vi "PPMSDR - Sweep control._Anilvi.vi"(0 "Scan control":cluster{"Priority":u16, "Scan name":u16}[](array[cluster])=[{"Priority"=0, "Scan name"=4}, {"Priority"=3, "Scan name"=0}, {"Priority"=1, "Scan name"=0}, {"Priority"=3, "Scan name"=0}] {"Scan name" items=["OFF", "Vsg1", "Vsg2", "Vsgw", "Vbg", "Field", "Temp", "MW_freq", "MW_amplitude"]; "Priority" items=["Priority 0", "Priority 1", "Priority 2", "Priority 3", "Priority 4", "Priority 5"]}, 1 "Scan parameters":T2(array[cluster])=[{"DAQ Channel"=2, "Label"="\nappliedVsg=", "Scaled low"=-0.1, "Scaled high"=0.6, "Start"=-2.0, "End"=2.0, "Step"=0.02, "Scale?"=FALSE}, {"DAQ Channel"=3, "Label"="\nappliedTemp=", "Scaled low"=-0.175, "Scaled high"=0.775, "Start"=0.35, "End"=0.05, "Step"=0.05, "Scale?"=FALSE}, {"DAQ Channel"=3, "Label"="\nappliedVbg=", "Scaled low"=-0.11, "Scaled high"=0.31, "Start"=-60000.0, "End"=0.0, "Step"=5000.0, "Scale?"=FALSE}, {"DAQ Channel"=3, "Label"="\nappliedField=", "Scaled low"=-0.060000000000000005, "Scaled high"=0.14, "Start"=-55000.0, "End"=0.0, "Step"=5000.0, "Scale?"=FALSE}] {"Step" format="%#_6p"; "End" format="%#_6p"; "Start" format="%#_6p"; "Scaled high" format="%#_6p"; "Scaled low" format="%#_6p"}, 2 "Channels: AO 2":T1={"AO amp (V)"=[0.005, 0.0, 0.0, 0.0], "AO DC (V)"=[0.0, 0.0, 0.0, 0.0], "AO f (Hz)"=[0.25, 0.25, 0.25, 0.25], "AO phi (deg)"=[0.0, 0.0, 0.0, 0.0], "function"=[enum."Sawtooth Wave", enum."Sine Wave", enum."Sine Wave", enum."Sine Wave"]} {"AO DC (V)" format="%#_6p"; "AO amp (V)" format="%#_6p"}, 3 "Comments":string="Backgate sweep from -2 to 2V in 15mV step\n 60 mK\n\nI1=0\nI2: Left wire 3/5:  1m, 0.2, sawtooth wave\nV1: 4-terminal Right wire 1/28\nV2: Cross-Barrier 4/1", 4 "Experiment folder name":string="05-backgatesweep_I1V_test") -> ()   [LabVIEW 2013]
uses:
  <userlib>/Levylab/DAQ-Lockin-SubVI/Lockin-4461_MultiChannel - IV 3.0 globals.vi
  Labview_Local/Lockin-4461_Multiple Inputs and Outputs_KH Folder/P/users1/Joe/Lockin-4461_3.0 4461-4462 Multichannel Folder/DAQ-Lockin-SubVI/Lock-in Globles Multiple Inputs and Outputs.vi
panel:
  in  "Additional action (indexing priority)":u16[](array[ring])=[5, 5, 5, 5] items=["Clear DAQ Tasks", "Check Temperature", "Check Field Value", "Wait", "Temp Below X", "Do Nothing"]
  in  "Enum":enum16{"IV", "lockin", "IV/lockin continuous B"}(ring)
  in  "Number of IV curves":i32=1
  # "Instructions: \n1, you can put multiple scan names in one priority.\n2 OFF has to put in last priority"
  # "if you use the lockin\nprogram remember to\nset BG/SG parameters in\n'lockin_Vsg_multichannel.vi'"
  # "Make sure Lockin is in REMOTE mode"
  # "0"
  # "1"
  # "2"
  # "3"
  # "4"
  # "5"
  # "6"
  # "7"
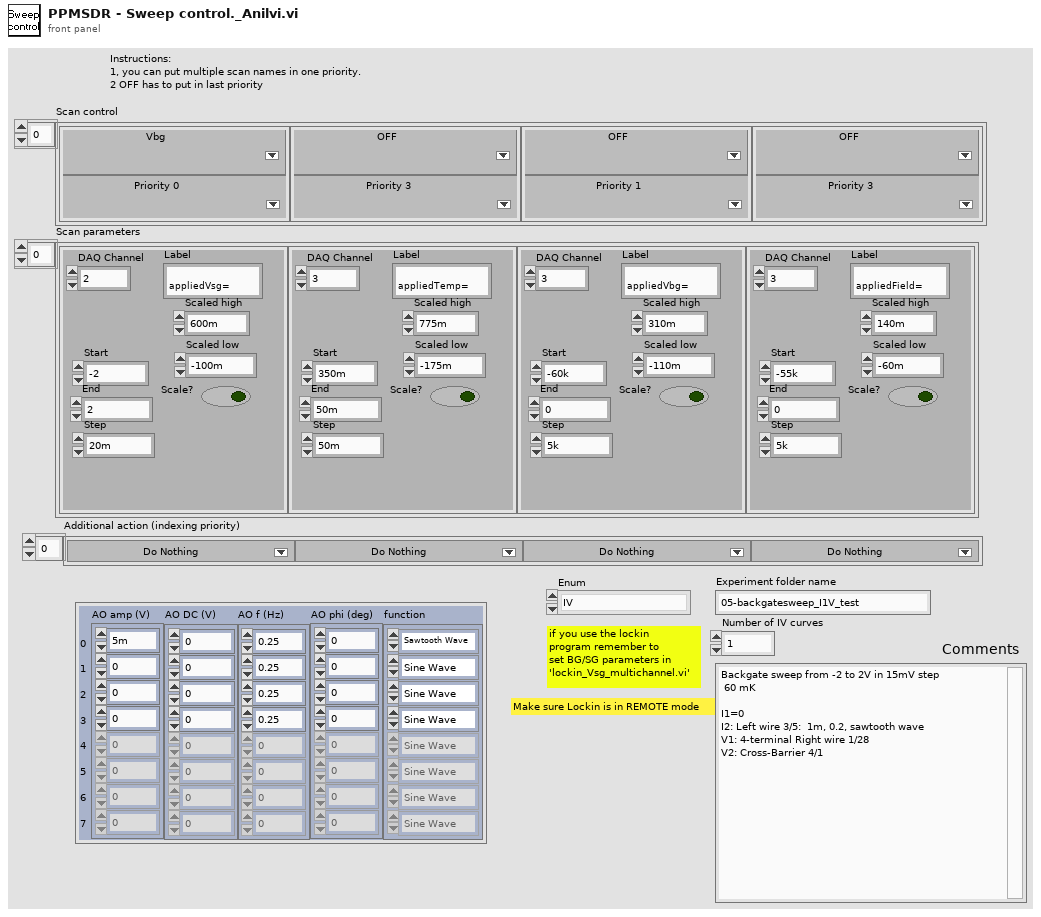
[diagram p1: front panel]
types:
  T1 = cluster{"AO amp (V)":dbl[], "AO DC (V)":dbl[], "AO f (Hz)":dbl[], "AO phi (deg)":dbl[], "function":enum16{"Sine Wave", "Triangle Wave", "Square Wave", "Sawtooth Wave"}[]}
  T2 = cluster{"DAQ Channel":i32, "Label":string, "Scaled low":dbl, "Scaled high":dbl, "Start":dbl, "End":dbl, "Step":dbl, "Scale?":bool}[]
  T3 = cluster{cluster{"DAQ Channel":i32, "Label":string, "Scaled low":dbl, "Scaled high":dbl, "Start":dbl, "End":dbl, "Step":dbl, "Scale?":bool}[]}[]
  T4 = cluster{cluster{"Priority":u16, "Scan name":u16}[]}[]
  T5 = cluster{cluster{"DAQ Channel":i32, "Label":string, "Scaled low":dbl, "Scaled high":dbl, "Start":dbl, "End":dbl, "Step":dbl, "Scale?":bool}[]}
  T6 = cluster{cluster{"Priority":u16, "Scan name":u16}[]}
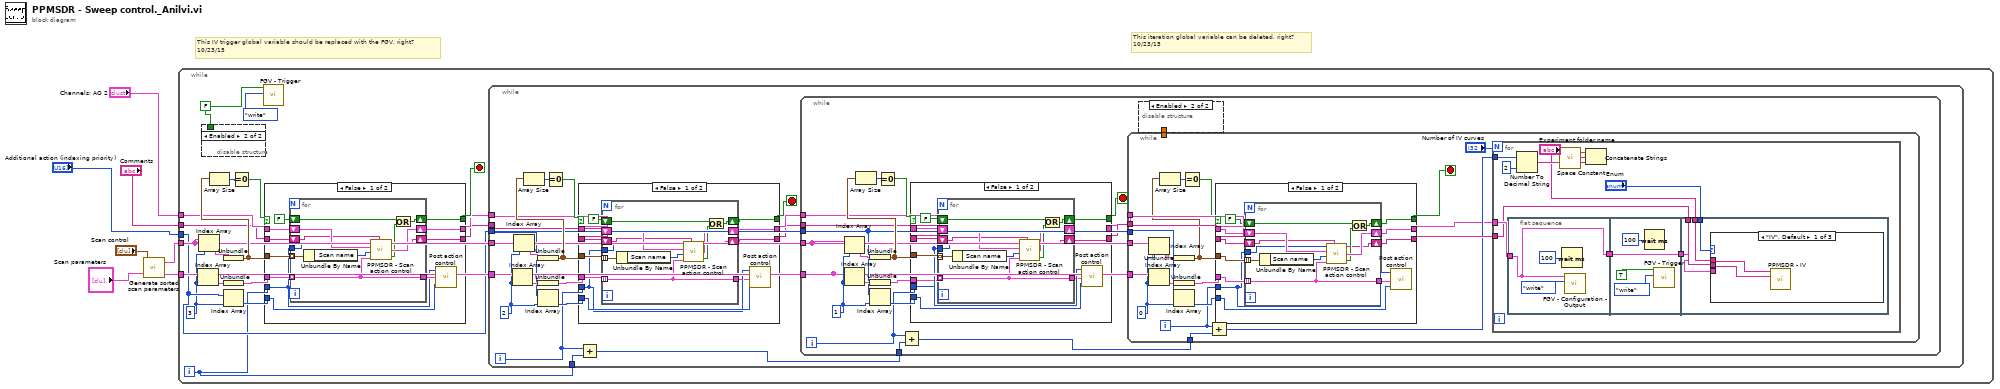
[diagram p0: block diagram]
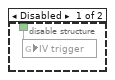
[diagram p2: hidden frame]
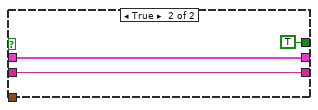
[diagram p3: hidden frame]
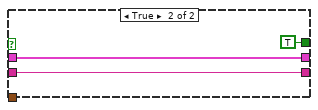
[diagram p4: hidden frame]
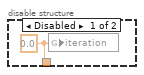
[diagram p5: hidden frame]
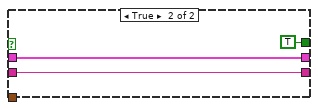
[diagram p6: hidden frame]
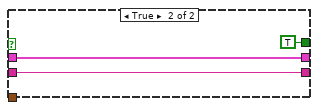
[diagram p7: hidden frame]
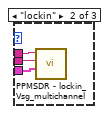
[diagram p8: hidden frame]
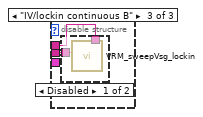
[diagram p9: hidden frame]
diagram:
  # "This IV trigger global variable should be replaced with the FGV, right?\n10/23/15"
  # "This iteration global variable can be deleted, right?\n10/23/15"
  n1 = call <userlib>:"Generate sorted scan parameters.vi"("Scan parameters"="Scan parameters", "Scan control"="Scan control") -> ("Sorted scan parameters"=w3:T3, "Sorted scan control"=w4:T4)
  n2 = while {
    tunnel: "Comments" -> [w14]
    tunnel: "Channels: AO 2" -> [w15]
    tunnel: w3 -> [w21]
    tunnel: w4 -> [w20]
    tunnel: "Additional action (indexing priority)" -> [w16]
    i -> [w10]
    stop <- w18 stop-if-true
    w8 = FALSE
    w11 = 3
    n3 = Index Array(array=w21, index=w11) -> (element=w22:T5)
    n4 = Index Array(array=w20, index=w11) -> (element=w19:T6)
    n5 = disable-structure shown="Enabled" {
      disable-tunnel: w8 -> [w27 _]
      frame Disabled {
        n6 = global write "Lock-in Globles Multiple Inputs and Outputs.vi" "IV trigger"(w27) -> ()
      }
      frame Enabled {
      }
    }
    n7 = Unbundle(w19) -> (w24:cluster{"Priority":u16, "Scan name":u16}[])
    n8 = Array Size(array=w24) -> (size(s)=w25:i32)
    n9 = Unbundle(w22) -> (w23:T2)
    n10 = Index Array(array=w16, index=w11) -> (element=w17:u16)
    n11 = Equal To 0?(x=w25) -> (x = 0?=w26:bool)
    n12 = call "FGV - Trigger.vi"("Function"=enum16{"write", "read"}."write", "Trigger"=w8) -> ()  [unwired: 4 in, 2 out]
    n13 = case shown="False" w26 {
      tunnel: w23 -> [w38 _]
      tunnel: [w37 w51] -> w13
      tunnel: [w36 w50] -> w12
      tunnel: [w30 TRUE ("Stop?")] -> w18
      tunnel: w24 -> [w35 _]
      tunnel: w10 -> [w32 _]
      tunnel: w17 -> [w33 _]
      tunnel: w15 -> [w29 w51]
      tunnel: w14 -> [w28 w50]
      frame False {
        n14 = for {
          tunnel: w35 -> [w49] mode=indexing
          tunnel: w38 -> [w46] mode=indexing
          tunnel: w32 -> [w43]
          shift-right: [w41] -> w37
          shift-left: w29 -> [w44]
          shift-right: [w39] -> w36
          shift-left: w28 -> [w42]
          tunnel: [w46] -> w34
          shift-right: [w47] -> w30
          shift-left: FALSE -> [w48]
          n15 = Unbundle By Name(w49) -> ("Scan name"=w45:u16)
          n16 = call <userlib>:"PPMSDR - Scan action control.vi"("Index"=w43, "Channels: AO"=w44, "Scan control"=w45, "Scan Parameters"=w46, "Comments"=w42) -> ("Comments out"=w39:string, "Channels: AO 2"=w41:T1, "Stop?"=w40:bool)
          n17 = Or(x=w48, y=w40) -> (x .or. y?=w47:bool)
        }
        n18 = call <userlib>:"Post action control.vi"("Action"=w33, "Scan Parameters"=w34, "Index"=w32) -> ()  [unwired: 1 out]
      }
      frame True {
      }
    }
    n19 = while {
      tunnel: w21 -> [w64]
      tunnel: w20 -> [w63]
      tunnel: w16 -> [w62]
      tunnel: w12 -> [w61]
      tunnel: w13 -> [w60]
      tunnel: w10 -> [w54]
      i -> [w55]
      stop <- w59 stop-if-true
      w56 = 2
      n20 = Index Array(array=w64, index=w56) -> (element=w70:T5)
      n21 = Index Array(array=w63, index=w56) -> (element=w71:T6)
      n22 = Unbundle(w71) -> (w68:cluster{"Priority":u16, "Scan name":u16}[])
      n23 = Array Size(array=w68) -> (size(s)=w66:i32)
      n24 = Unbundle(w70) -> (w69:T2)
      n25 = Index Array(array=w62, index=w56) -> (element=w67:u16)
      n26 = Equal To 0?(x=w66) -> (x = 0?=w65:bool)
      n27 = case shown="False" w65 {
        tunnel: w69 -> [w77 _]
        tunnel: w60 -> [w80 w96]
        tunnel: w61 -> [w79 w95]
        tunnel: [w74 w96] -> w58
        tunnel: [w73 w95] -> w57
        tunnel: [w75 TRUE ("Stop?")] -> w59
        tunnel: w68 -> [w78 _]
        tunnel: w55 -> [w76 _]
        tunnel: w67 -> [w82 _]
        frame False {
          n28 = for {
            tunnel: w78 -> [w93] mode=indexing
            tunnel: w77 -> [w90] mode=indexing
            tunnel: w76 -> [w87]
            shift-right: [w85] -> w74
            shift-left: w80 -> [w88]
            shift-right: [w83] -> w73
            shift-left: w79 -> [w86]
            tunnel: [w90] -> w72
            shift-right: [w91] -> w75
            shift-left: FALSE -> [w92]
            n29 = Unbundle By Name(w93) -> ("Scan name"=w89:u16)
            n30 = call <userlib>:"PPMSDR - Scan action control.vi"("Index"=w87, "Channels: AO"=w88, "Scan control"=w89, "Scan Parameters"=w90, "Comments"=w86) -> ("Comments out"=w83:string, "Channels: AO 2"=w85:T1, "Stop?"=w84:bool)
            n31 = Or(x=w92, y=w84) -> (x .or. y?=w91:bool)
          }
          n32 = call <userlib>:"Post action control.vi"("Action"=w82, "Scan Parameters"=w72, "Index"=w76) -> ()  [unwired: 1 out]
        }
        frame True {
        }
      }
      n33 = Add(x=w55, y=w54) -> (x+y=w53:i32)
      n34 = while {
        tunnel: w58 -> [w98]
        tunnel: w57 -> [w108]
        tunnel: w63 -> [w107]
        tunnel: w64 -> [w97]
        tunnel: w62 -> [w106]
        tunnel: w53 -> [w100]
        i -> [w101]
        stop <- w103 stop-if-true
        w102 = 1
        n35 = Index Array(array=w107, index=w102) -> (element=w109:T6)
        n36 = Index Array(array=w97, index=w102) -> (element=w110:T5)
        n37 = Unbundle(w109) -> (w112:cluster{"Priority":u16, "Scan name":u16}[])
        n38 = Array Size(array=w112) -> (size(s)=w114:i32)
        n39 = Unbundle(w110) -> (w111:T2)
        n40 = Index Array(array=w106, index=w102) -> (element=w113:u16)
        n41 = Equal To 0?(x=w114) -> (x = 0?=w115:bool)
        n42 = Add(x=w101, y=w100) -> (x+y=w99:i32)
        n43 = case shown="False" w115 {
          tunnel: w111 -> [w122 _]
          tunnel: w98 -> [w126 w142]
          tunnel: w108 -> [w125 w141]
          tunnel: [w120 w142] -> w104
          tunnel: [w119 w141] -> w105
          tunnel: [w121 TRUE ("Stop?")] -> w103
          tunnel: w112 -> [w124 _]
          tunnel: w101 -> [w123 _]
          tunnel: w113 -> [w128 _]
          frame False {
            n44 = for {
              tunnel: w124 -> [w139] mode=indexing
              tunnel: w122 -> [w136] mode=indexing
              tunnel: w123 -> [w133]
              shift-right: [w131] -> w120
              shift-left: w126 -> [w134]
              shift-right: [w129] -> w119
              shift-left: w125 -> [w132]
              tunnel: [w136] -> w118
              shift-right: [w137] -> w121
              shift-left: FALSE -> [w138]
              n45 = Unbundle By Name(w139) -> ("Scan name"=w135:u16)
              n46 = call <userlib>:"PPMSDR - Scan action control.vi"("Index"=w133, "Channels: AO"=w134, "Scan control"=w135, "Scan Parameters"=w136, "Comments"=w132) -> ("Comments out"=w129:string, "Channels: AO 2"=w131:T1, "Stop?"=w130:bool)
              n47 = Or(x=w138, y=w130) -> (x .or. y?=w137:bool)
            }
            n48 = call <userlib>:"Post action control.vi"("Action"=w128, "Scan Parameters"=w118, "Index"=w123) -> ()  [unwired: 1 out]
          }
          frame True {
          }
        }
        n49 = disable-structure shown="Enabled" {
          disable-tunnel: [w117 _] -> w116
          frame Disabled {
            w117 = 0.0 ("iteration")
            n50 = global write "Lockin-4461_MultiChannel - IV 3.0 globals.vi" "iteration"(w117) -> ()
          }
          frame Enabled {
          }
        }
        n51 = while {
          tunnel: w107 -> [w161]
          tunnel: w97 -> [w160]
          tunnel: w104 -> [w156]
          tunnel: w105 -> [w155]
          tunnel: w106 -> [w151]
          tunnel: w116 -> [_]
          tunnel: w99 -> [w145]
          i -> [w146]
          stop <- w153 stop-if-true
          w148 = 0
          n52 = Index Array(array=w161, index=w148) -> (element=w159:T6)
          n53 = Index Array(array=w160, index=w148) -> (element=w158:T5)
          n54 = Unbundle(w159) -> (w152:cluster{"Priority":u16, "Scan name":u16}[])
          n55 = Array Size(array=w152) -> (size(s)=w150:i32)
          n56 = Unbundle(w158) -> (w157:T2)
          n57 = Index Array(array=w151, index=w148) -> (element=w147:u16)
          n58 = Equal To 0?(x=w150) -> (x = 0?=w149:bool)
          n59 = Add(x=w146, y=w145) -> (x+y=w144:i32)
          n60 = case shown="False" w149 {
            tunnel: w157 -> [w168 _]
            tunnel: w156 -> [w171 w187]
            tunnel: w155 -> [w170 w186]
            tunnel: [w165 w187] -> w143
            tunnel: [w164 w186] -> w154
            tunnel: [w166 TRUE ("Stop?")] -> w153
            tunnel: w152 -> [w169 _]
            tunnel: w146 -> [w167 _]
            tunnel: w147 -> [w173 _]
            frame False {
              n61 = for {
                tunnel: w169 -> [w184] mode=indexing
                tunnel: w168 -> [w181] mode=indexing
                tunnel: w167 -> [w178]
                shift-right: [w176] -> w165
                shift-left: w171 -> [w179]
                shift-right: [w174] -> w164
                shift-left: w170 -> [w177]
                tunnel: [w181] -> w163
                shift-right: [w182] -> w166
                shift-left: FALSE -> [w183]
                n62 = Unbundle By Name(w184) -> ("Scan name"=w180:u16)
                n63 = call <userlib>:"PPMSDR - Scan action control.vi"("Index"=w178, "Channels: AO"=w179, "Scan control"=w180, "Scan Parameters"=w181, "Comments"=w177) -> ("Comments out"=w174:string, "Channels: AO 2"=w176:T1, "Stop?"=w175:bool)
                n64 = Or(x=w183, y=w175) -> (x .or. y?=w182:bool)
              }
              n65 = call <userlib>:"Post action control.vi"("Action"=w173, "Scan Parameters"=w163, "Index"=w167) -> ()  [unwired: 1 out]
            }
            frame True {
            }
          }
          n66 = for {
            N: "Number of IV curves" -> [_]
            tunnel: w143 -> [w197]
            tunnel: w154 -> [w191]
            tunnel: w144 -> [w195]
            n67 = flat-sequence {
              tunnel: w197 -> [w198]
              tunnel: [w198] -> w188
              tunnel: [w201] -> w189
              tunnel: w188 -> [w201]
              tunnel: "Enum" -> [w208]
              tunnel: w191 -> [w207]
              tunnel: "Experiment folder name" -> [w206]
              tunnel: w189 -> [w205]
              frame #0 {
                n68 = Wait (ms)(milliseconds to wait=u32 100) -> ()  [unwired: 1 out]
                n69 = call "FGV - Configuration - Output.vi"("Function"=enum16{"write", "read"}."write", "Channels: AO"=w198) -> ()  [unwired: 4 in, 2 out]
              }
              frame #1 {
                n70 = Wait (ms)(milliseconds to wait=u32 100) -> ()  [unwired: 1 out]
                n71 = call "FGV - Trigger.vi"("Function"=enum16{"write", "read"}."write", "Trigger"=TRUE) -> ()  [unwired: 4 in, 2 out]
              }
              frame #2 {
                n72 = case shown="\"IV\", Default" w208 {
                  tunnel: w207 -> [w209 w212 w214]
                  tunnel: w206 -> [w210 w213 w215]
                  tunnel: w205 -> [_ w211 _]
                  frame "IV", Default {
                    n73 = call "PPMSDR - IV.vi"("Notes"=w209, "Experiment folder name"=w210) -> ()  [unwired: 10 in]
                  }
                  frame "lockin" {
                    n74 = call "PPMSDR - lockin_Vsg_multichannel.vi"("Channels: AO"=w211, "Comments"=w212, "ITX folder"=w213) -> ()  [unwired: 9 in]
                  }
                  frame "IV/lockin continuous B" {
                    n75 = disable-structure shown="Disabled" {
                      disable-tunnel: w215 -> [w217 _]
                      disable-tunnel: w214 -> [w216 _]
                      frame Disabled {
                        n76 = call "VRM_sweepVsg_lockin.vi"("Comments"=w216, "ITX folder"=w217) -> ()  [unwired: 7 in, 1 out]
                      }
                      frame Enabled {
                      }
                    }
                  }
                }
              }
            }
            n77 = Number To Decimal String(number=w195, width (-)=i16 2) -> (decimal integer string=w194:string)
            n78 = call <vilib>:"Space Constant.vi"() -> ("String"=w193:string)
            n79 = Concatenate Strings("Experiment folder name", w193, w194) -> ()  [unwired: 1 out]
          }
        }
      }
    }
  }
